vi "Load Parameterized Executive.vi"(5 "Path Builder":refnum<class "IPath Builder.lvclass">, 6 "Folder":path, 7 "Compatibility Helper":refnum<class "ICompatibility Helper.lvclass">, 8 "error in (no error)":errorcluster, 9 "Persistence in":refnum<class "IPersist.lvclass">, 10 "Test Executive":refnum<class "ITest Executive.lvclass">, 11 "Test Executive in":refnum<class "Test Executive.lvclass">) -> (0 "error out":errorcluster, 3 "Test Executive out":refnum<class "Test Executive.lvclass">)   [LabVIEW 2017, in "Test Executive.lvlib" / "Test Executive.lvclass"]
uses:
  <vilib>/gpm_packages/@cs/test-executive/Source/Test Executive/TestExecutive/Test Executive.lvclass
  <vilib>/gpm_packages/@cs/test-executive/Source/Test Executive/ITestExecutive/ITest Executive.lvclass
  <vilib>/gpm_packages/@cs/persistence/source/IPersist/IPersist.lvclass
  <vilib>/gpm_packages/@cs/test-executive/Source/Path Builder/IPath Builder/IPath Builder.lvclass
  <vilib>/gpm_packages/@cs/test-executive/Source/Compatibility Helper/ICompatibility Helper.lvclass
  <vilib>/gpm_packages/@cs/test-executive/Source/Test Executive/TestExecutive Ref/TestExecutive Ref.lvclass
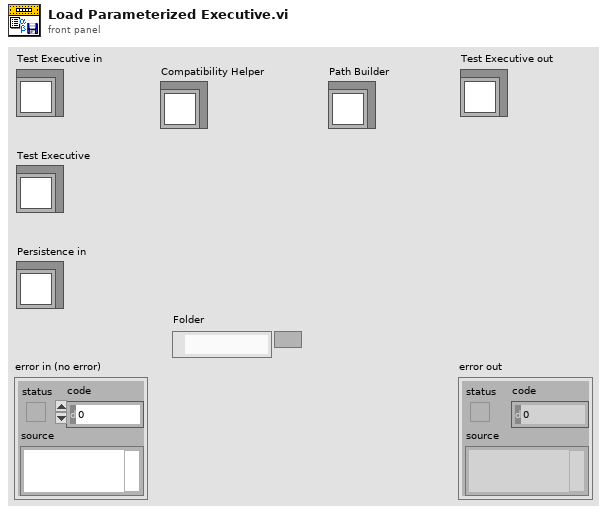
[diagram p1: front panel]
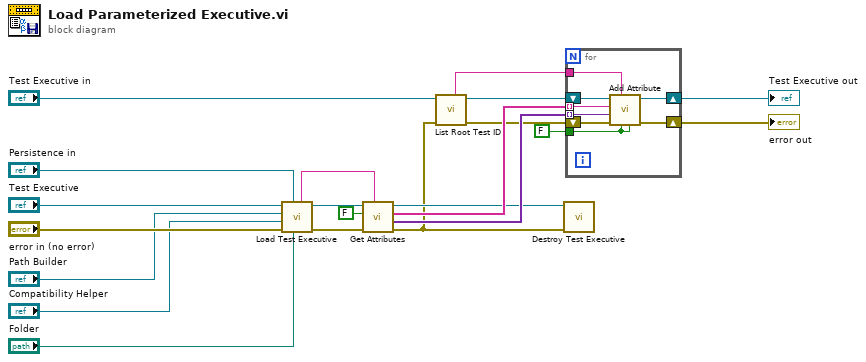
[diagram p0: block diagram]
diagram:
  n1 = call <vilib>:"Load Test Executive.vi"("Folder"="Folder", "Persistence in"="Persistence in", "error in (no error)"="error in (no error)", "Compatibility Helper"="Compatibility Helper", "Path Builder"="Path Builder", "Test Executive"="Test Executive") -> ("error out"=w14:errorcluster, "Test Executive Ref out"=w15:refnum<data-value>, "Root ID"=w13:string)  [unwired: 3 in]
  n2 = call <vilib>:"Get Attributes.vi"("Test ID"=w13, "error in (no error)"=w14, "Include Private?"=FALSE, "Test Executive Ref"=w15) -> ("error out"=w1:errorcluster, "Attributes"=w6:variant[], "Attribute Names out"=w7:string[], "Test Executive Ref out"=w2:refnum<data-value>)  [unwired: 2 in, 2 out]
  n3 = call-dynamic "List Root Test ID.vi"("error in (no error)"=w1, "Test Executive in"="Test Executive in") -> ("error out"=w4:errorcluster, "Test Executive out"=w10:refnum<class "Test Executive.lvclass">, "Root ID"=w8:string)  [unwired: 5 in, 2 out]
  n4 = call <vilib>:"Destroy Test Executive.vi"("error in (no error)"=w1, "Test Executive Ref"=w2) -> ()  [unwired: 9 in, 1 out]
  n5 = for {
    tunnel: w8 -> [w27]
    shift-right: [w28] -> w9
    shift-left: w10 -> [w29]
    tunnel: w7 -> [w26] mode=indexing
    tunnel: w6 -> [w25] mode=indexing
    tunnel: FALSE -> [w24]
    shift-right: [w22] -> w3
    shift-left: w4 -> [w23]
    n6 = call-dynamic "Add Attribute.vi"("Private?"=w24, "Pointer?"=w24, "ID"=w27, "error in (no error)"=w23, "Attribute"=w25, "Attribute Name"=w26, "Test Executive in"=w29) -> ("error out"=w22:errorcluster, "Test Executive out"=w28:refnum<class "Test Executive.lvclass">)  [unwired: 1 in, 2 out]
  }
  "error out" <- w3
  "Test Executive out" <- w9
